vi "Wait.vi"   [LabVIEW 2014, in "niInstr Streaming v1 Host.lvlib"]
uses:
  <instrlib>/_niInstr/Streaming/v1/Host/niInstr Streaming v1 Host.lvlib
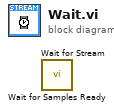
[diagram p0: block diagram]
diagram:
  n1 = call <instrlib>:"Wait for Samples Ready.vi"() -> ()  [unwired: 9 in, 3 out]
  n2 = call <instrlib>:"Wait for Stream.vi"() -> ()  [unwired: 8 in, 4 out]
